vi "ATE_BSE_Event Queue FGV.vi"(6 "Operations":T1, 8 "error in (no error)":errorcluster, 11 "Queue name":string) -> (0 "error out":errorcluster, 3 "queue out":refnum<queue>)   [LabVIEW 2021]
uses:
  Controls/ATE_BSE_Queue_Operations.ctl
  Controls/ATE_BSE_Event_type_def.ctl
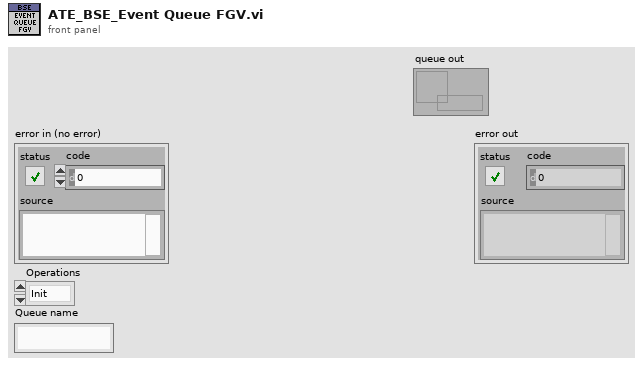
[diagram p1: front panel]
types:
  T1 = typedef "ATE_BSE_Queue_Operations.ctl" = enum16{"Init", "Get Queue", "Flush", "Close"}
  T2 = typedef "ATE_BSE_Event_type_def.ctl" = enum16{"Initialize", "Configure", "Ip Simulation", "UE-Display", "IMS", "Sim Configurations", "ECall", "Exit", "Error"}
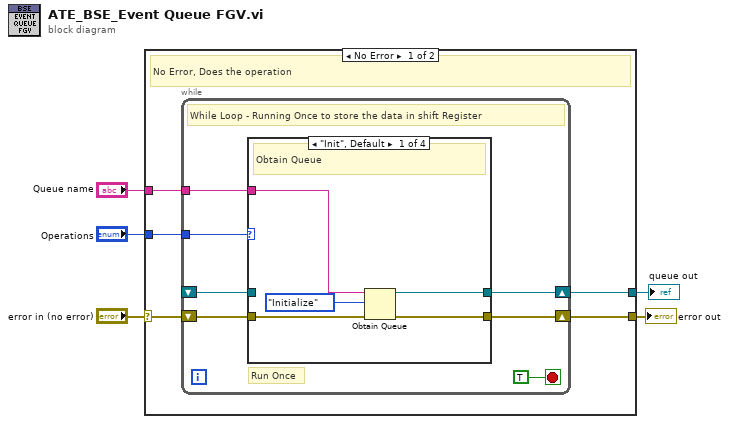
[diagram p0: block diagram]
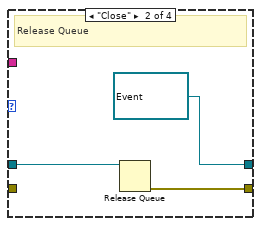
[diagram p2: hidden frame]
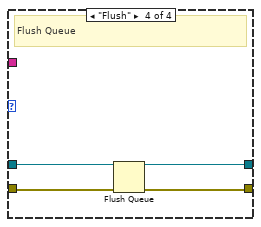
[diagram p4: hidden frame]
diagram:
  n1 = case shown="No Error" "error in (no error)" {
    selector: "error in (no error)" -> [w9 w32]
    tunnel: [w8 w32] -> w2
    tunnel: "Operations" -> [w10 _]
    tunnel: "Queue name" -> [w7 _]
    tunnel: [w6 _] -> w1
    frame No Error {
      # "No Error, Does the operation"
      n2 = while {
        tunnel: w10 -> [w16]
        shift-right: [w14] -> w8
        shift-left: w9 -> [w15]
        tunnel: w7 -> [w13]
        shift-right: [w12] -> w6
        shift-left: _ -> [w11]
        stop <- TRUE stop-if-true
        # "Run Once"
        # "While Loop - Running Once to store the data in shift Register"
        n3 = case shown="\"Init\", Default" w16 {
          tunnel: w15 -> [w22 _ w26 w30]
          tunnel: [w21 w24 w26 w29] -> w14
          tunnel: w13 -> [w20 _ _ _]
          tunnel: [w19 w23 w27 w28] -> w12
          tunnel: w11 -> [_ w25 w27 w31]
          frame "Init", Default {
            # "Obtain Queue"
            n4 = Obtain Queue(name (unnamed)=w20, element data type=ATE_BSE_Event_type_def."Initialize" ("Event"), error in (no error)=w22) -> (queue out=w19:refnum<queue>, error out=w21:errorcluster)  [unwired: 2 in, 1 out]
          }
          frame "Close" {
            w23 = refnum<queue> refnum items=["Initialize", "Configure", "Ip Simulation", "UE-Display", "IMS", "Sim Configurations", "ECall", "Exit", "Error"] ("queue out")
            # "Release Queue"
            n5 = Release Queue(queue=w25) -> (error out=w24:errorcluster)  [unwired: 2 in, 2 out]
          }
          frame "Get Queue" {
            # "Enqueue the Element into the Queue"
          }
          frame "Flush" {
            # "Flush Queue"
            n6 = Flush Queue(queue=w31, error in (no error)=w30) -> (queue out=w28:refnum<queue>, error out=w29:errorcluster)  [unwired: 1 out]
          }
        }
      }
    }
    frame Error {
      # "Gives out the next state as Error"
      # "Error, Does nothing"
    }
  }
  "error out" <- w2
  "queue out" <- w1
